vi "ROS_Topic_Write_Primitive.vi"(2 "Msg in":string, 3 "ROS in":T1) -> (1 "ROS out":T1)   [LabVIEW 2013]
doc: "Writes the data to background server when publishing data or sending service calls. Implemented in ROS_Topic_Write and ROS_Topic_Write_Continuous."
uses:
  SubVIs/_ROSControl.ctl
  SubVIs/_ROSDirection.ctl
panel:
  out "resulting string":string
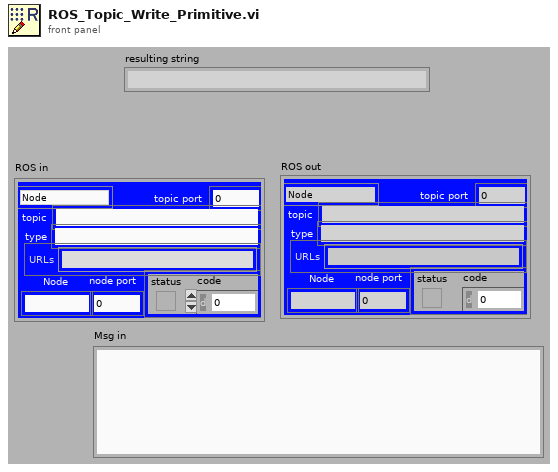
[diagram p1: front panel]
types:
  T1 = typedef "_ROSControl.ctl" = cluster{"topic port":u16, "Node":string, "topic":string, "type":string, "node port":u32, "error ":errorcluster, "Direction":T2, "APIs":string[]}
  T2 = typedef "_ROSDirection.ctl" = enum16{"Node", "Publisher", "Subscriber", "Service Client"}
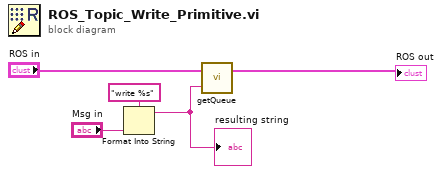
[diagram p0: block diagram]
diagram:
  n1 = Format Into String(format string="write %s" ("name (unnamed)"), "Msg in") -> (resulting string=w1:string)  [unwired: 2 in, 1 out]
  "resulting string" <- w1
  n2 = call "getQueue.vi"("queue msg"=w1, "ROS in"="ROS in") -> ("ROS out"=→"ROS out":T1)  [unwired: 1 in]
